vi "Auto Griddy Score v2_wrapper.vi"() -> ()   [LabVIEW 2020]
uses:
  <vilib>/Rock Robotics/WPI/Framework/Command Status Info.ctl
  <vilib>/Rock Robotics/WPI/Framework/Completion Status.ctl
  <vilib>/Rock Robotics/WPI/Framework/Completion Notifier.ctl
  intake sub/Implementation/Typedef/intake typedef.ctl
  Implementation/Typedefs/Teleop Manipulator Commands.ctl
panel:
  out "Command Info Out":T1
  in  "Griddy Command":T4
  in  "intake modes":T5
  in  "Command Info In":T1
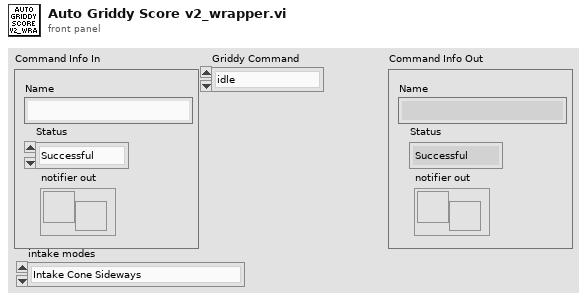
[diagram p1: front panel]
types:
  T1 = typedef "Command Status Info.ctl" = cluster{"Name":string, "Status":T2, "notifier out":T3}
  T2 = typedef "Completion Status.ctl" = enum16{"Successful", "Aborted", "Incomplete"}
  T3 = typedef "Completion Notifier.ctl" = refnum<notifier>
  T4 = typedef "Teleop Manipulator Commands.ctl" = enum16{"idle", "intake cone sideways", "intake cone upright", "intake cone feeder", "intake cube feeder", "intake cube", "score low cone", "score low cube", "score mid cone", "score mid cube", "score high cone", "score high cube", "score mid cone up"}
  T5 = typedef "intake typedef.ctl" = enum16{"Intake Cone Sideways", "Intake Cone Upright", "Intake Cube", "Outtake/Score", "Shoot"}
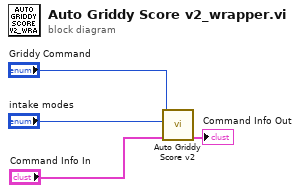
[diagram p0: block diagram]
diagram:
  n1 = call "Auto Griddy Score v2.vi"("Command Info In"="Command Info In", "intake modes"="intake modes", "Griddy Command"="Griddy Command") -> ("Command Info Out"=→"Command Info Out":T1)  [unwired: 8 in]
